vi "Requests.vi"(8 "error in (no error)":errorcluster, 9 "write enable":bool=TRUE, 11 "ICPCON ET-7017 in":refnum<class "ICPCON ET-7017-10.lvclass">) -> (0 "error out":errorcluster, 3 "ICPCON ET-7017 out":refnum<class "ICPCON ET-7017-10.lvclass">)   [LabVIEW 2021, in "ICPCON ET-7017-10.lvclass"]
uses:
  ICPCON ET-7017-10.lvclass
  D:/my_projects/projects/Algorithms/Labview/21/Modbus_v2/MB/Modbus Master CR.lvclass
  D:/my_projects/projects/Algorithms/Labview/21/Modbus_v121c/Network Protocol/Network Master/Network Master.lvclass
  MB/Modbus Master CR.lvclass/Modbus Master CR.ctl
  Modbus Data Unit/Modbus Data Unit.lvclass/Modbus Data Unit.ctl
  Network Protocol.lvclass/Network Protocol.ctl
  Network Master/Network Master.lvclass/Network Master.ctl
  Master Function Definition/Read Input Registers Request.vi
  Master Function Definition/Read Input Registers Response.vi
  Network Master/Read write Master.vi
  Modbus Data Unit/Construct PDU.vi
  Utility/Bytes to U16s.vi
  Master Function Definition/Function code mismatch error.vi
  Data Model/Error Generator.vi
  Modbus Data Unit/Deconstruct PDU.vi
  Read Transmission Data Unit.vi
  Network Master/Network Master.lvclass
  D:/my_projects/projects/Algorithms/Labview/21/Modbus_v121c/Network Protocol/Network Protocol.lvclass
  Modbus Data Unit/Modbus Data Unit.lvclass
  Data Model/Device Data Model.lvclass
  Transmission Data Unit/Transmission Data Unit.lvclass
  ICPCON ET-7017-10.lvclass/ICPCON ET-7017-10.ctl
  MB/Modbus Master CR.lvclass
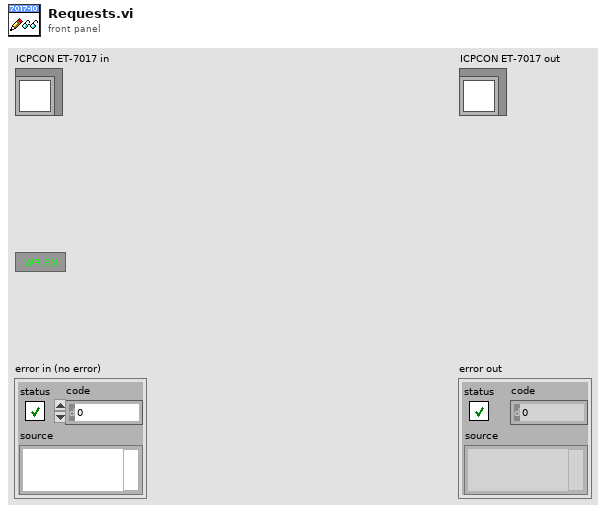
[diagram p1: front panel]
types:
  T1 = typedef "Modbus Master CR.lvclass/N channel.ctl" = cluster{"N DI channel":u16, "N DO channel":u16, "N AI channel":u16, "N AO channel":u16}
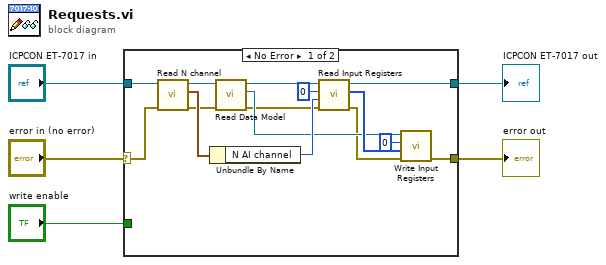
[diagram p0: block diagram]
diagram:
  n1 = case shown="No Error" "error in (no error)" {
    selector: "error in (no error)" -> [w13 w22]
    tunnel: [w9 w22] -> w3
    tunnel: [w6 w21] -> w4
    tunnel: "ICPCON ET-7017 in" -> [w15 w21]
    tunnel: "write enable" -> [_ _]
    frame No Error {
      n2 = call "Read N channel.vi"("error in (no error)"=w13, "MB_v2 in"=w15) -> ("error out"=w12:errorcluster, "N channel"=w17:T1, "MB_v2 out"=w14:refnum<class "ICPCON ET-7017-10.lvclass">)  [unwired: 7 in]
      n3 = Unbundle By Name(w17) -> ("N AI channel"=w16:u16)
      n4 = call "Read Data Model.vi"("error in (no error)"=w12, "MB_TCP in"=w14) -> ("error out"=w7:errorcluster, "Data Model"=w11:refnum<class "Device Data Model.lvclass">, "MB_TCP out"=w8:refnum<class "ICPCON ET-7017-10.lvclass">)  [unwired: 7 in]
      n5 = call "Read Input Registers.vi"("error in (no error)"=w7, "number of input registers"=w16, "starting address"=u16 0, "Modbus master in"=w8) -> ("error out"=w10:errorcluster, "register values"=w19:u16[], "Modbus master out"=w6:refnum<class "ICPCON ET-7017-10.lvclass">)  [unwired: 5 in]
      n6 = call-dynamic "Write Input Registers.vi"("error in (no error)"=w10, "register values"=w19, "starting address"=u16 0, "Device Data Model in"=w11) -> ("error out"=w9:errorcluster)  [unwired: 6 in, 1 out]
    }
    frame Error {
    }
  }
  "error out" <- w3
  "ICPCON ET-7017 out" <- w4
